vi "защита  (SubVI).vi"(6 "N":i32, 9 "m":dbl, 10 "k":dbl, 11 "n":dbl) -> (2 "Array":dbl[](array[numeric]), 3 "Array 2":dbl[](array[numeric]))   [LabVIEW 2012]
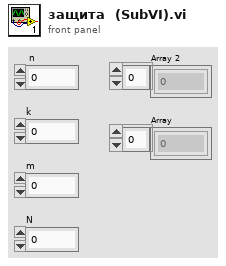
[diagram p1: front panel]
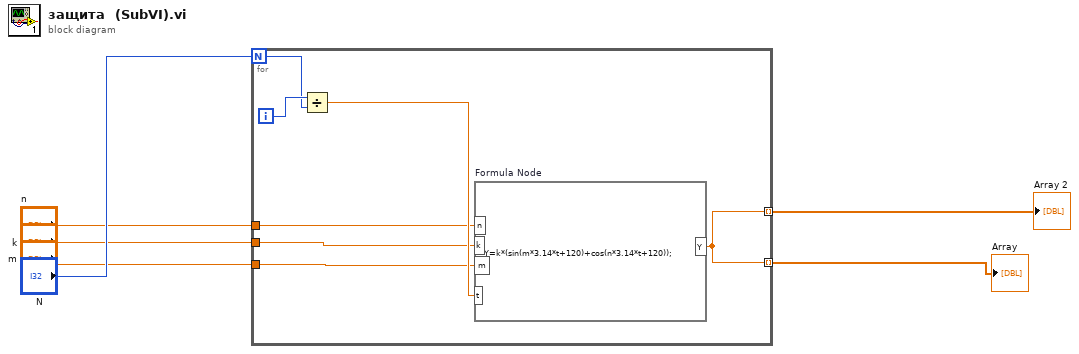
[diagram p0: block diagram]
diagram:
  n1 = for {
    N: "N" -> [w12]
    tunnel: [w10] -> w1 mode=indexing
    tunnel: [w10] -> w2 mode=indexing
    tunnel: "n" -> [w9]
    tunnel: "k" -> [w8]
    tunnel: "m" -> [w7]
    i -> [w13]
    n2 = Divide(x=w13, y=w12) -> (x/y=w11:dbl)
    n3 = formula code="Y=k*(sin(m*3.14*t+120)+cos(n*3.14*t+120));"("k"=w8, "m"=w7, "t"=w11, "n"=w9) -> ("Y"=w10:dbl)
  }
  "Array" <- w2
  "Array 2" <- w1
